vi "LED BASIC-1.vi"() -> ()   [LabVIEW 2018]
panel:
  out "Indicator":bool
  in  "Control":bool
  # "LED BASIC"
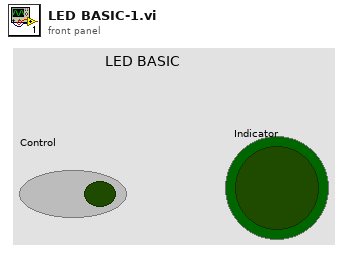
[diagram p1: front panel]
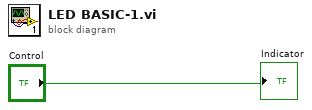
[diagram p0: block diagram]
diagram:
  "Indicator" <- "Control"
